vi "String_parsingV5.2.vi"(0 "input string":string) -> (1 "sekundes":i32, 2 "minute":i32, 3 "V1":i32[](array[numeric]), 4 "V3":i32[](array[numeric]), 5 "V2":i32[](array[numeric]), 6 "hour":i32)   [LabVIEW 2014]
panel:
  out "size(s)":i32
  out "input test":u8[](array[numeric])
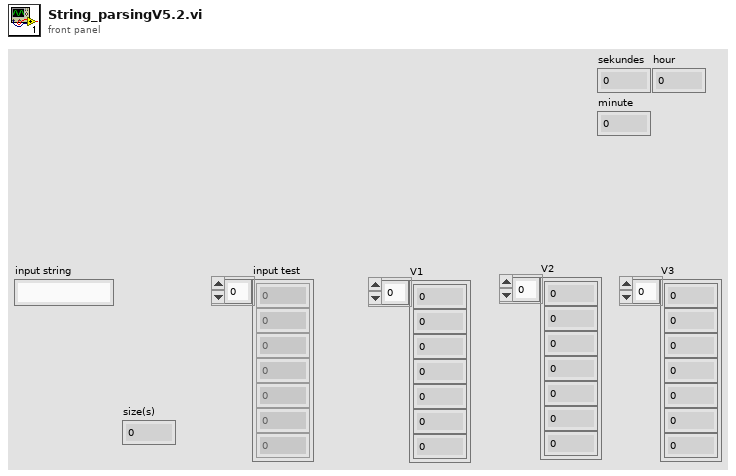
[diagram p1: front panel]
types:
  T1 = typedef "LVDateTimeRec.ctl" = cluster{"fractional second":dbl, "second":i32, "minute":i32, "hour":i32, "day of month":i32, "month":i32, "year":i32, "day of week":i32, "day of year":i32, "DST":i32}
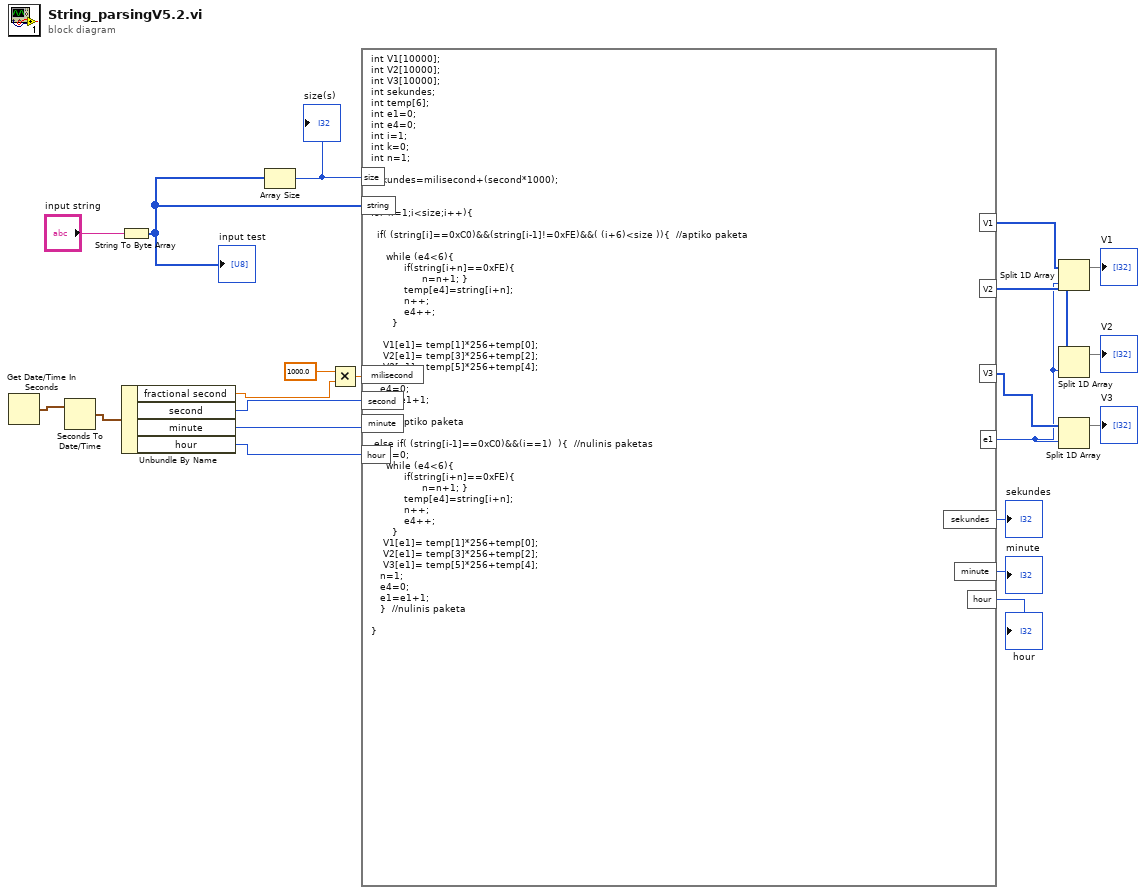
[diagram p0: block diagram]
diagram:
  n1 = Get Date/Time In Seconds() -> (seconds since 1Jan1904=w11:timestamp)
  n2 = Seconds To Date/Time(time stamp (now)=w11) -> (date time rec=w10:T1)  [unwired: 1 in]
  n3 = String To Byte Array(string="input string") -> (unsigned byte array=w21:u8[])
  "input test" <- w21
  n4 = Unbundle By Name(w10) -> ("fractional second"=w6:dbl, "second"=w9:i32, "minute"=w8:i32, "hour"=w7:i32)
  n5 = Array Size(array=w21) -> (size(s)=w20:i32)
  "size(s)" <- w20
  n6 = Multiply(x=1000.0, y=w6) -> (x*y=w4:dbl)
  n7 = formula code="int V1[10000];\nint V2[10000];\nint V3[10000];\nint sekundes;\nint temp[6];\nint e1=0;\nint e4=0;\nint i=1;\nint k=0;\nint n=1;\n\nsekundes=milisecond+(second*1000);\n\n\nfor (i=1;i<size;i++){\n \n  if( (string[i]==0xC0)&&(string[i-1]!=0xFE)&&( (i+6)<size )){  //aptiko paketa\n\n     while (e4<6){\n           if(string[i+n]==0xFE){\n                 n=n+1; }\n           temp[e4]=string[i+n];\n           n++; \n           e4++;\n       }\n   \n    V1[e1]= temp[1]*256+temp[0];\n    V2[e1]= temp[3]*256+temp[2];\n    V3[e1]= temp[5]*256+temp[4];\n   n=1;\n   e4=0;\n   e1=e1+1;\n   \n   }  //aptiko paketa\n\n else if( (string[i-1]==0xC0)&&(i==1)  ){  //nulinis paketas\n     n=0;\n     while (e4<6){\n           if(string[i+n]==0xFE){\n                 n=n+1; }\n           temp[e4]=string[i+n];\n           n++; \n           e4++;\n       }\n    V1[e1]= temp[1]*256+temp[0];\n    V2[e1]= temp[3]*256+temp[2];\n    V3[e1]= temp[5]*256+temp[4];\n   n=1;\n   e4=0;\n   e1=e1+1;\n   }  //nulinis paketa\n\n}"("string"=w21, "size"=w20, "milisecond"=w4, "second"=w9, "minute"=w8, "hour"=w7) -> ("V1"=w18:i32[], "V2"=w14:i32[], "V3"=w13:i32[], "e1"=w12:i32, "sekundes"=→"sekundes":i32, "minute"=→"minute":i32, "hour"=→"hour":i32)
  n8 = Split 1D Array(array=w18, index=w12) -> (first subarray=→"V1":i32[])  [unwired: 1 out]
  n9 = Split 1D Array(array=w14, index=w12) -> (first subarray=→"V2":i32[])  [unwired: 1 out]
  n10 = Split 1D Array(array=w13, index=w12) -> (first subarray=→"V3":i32[])  [unwired: 1 out]
